vi "Cursor Release.vi"(6 "Control Ref Queue":T1, 8 "error in (no error)":errorcluster, 11 "2D Plot.lvclass in":refnum<class "2D Plot.lvclass">) -> (0 "error out":errorcluster, 3 "2D Plot.lvclass out":refnum<class "2D Plot.lvclass">)   [LabVIEW 2017, in "2D Plot.lvclass"]
uses:
  <vilib>/Math Plots/2D Math Plots/2D Plot/2D Plot/2D Plot.lvclass
  <vilib>/Math Plots/2D Math Plots/2D Plot/Action String/2DMathPlot Ctrl Act Queue.ctl
  <vilib>/Math Plots/2D Math Plots/2D Plot/Action String/2DMathPlot Ctrl Act Cluster.ctl
  <vilib>/Math Plots/2D Math Plots/2D Plot/Action String/2DMathPlot State Class.ctl
  <vilib>/Math Plots/2D Math Plots/2D Plot/2D Plot/2D Plot.lvclass/2D Plot.ctl
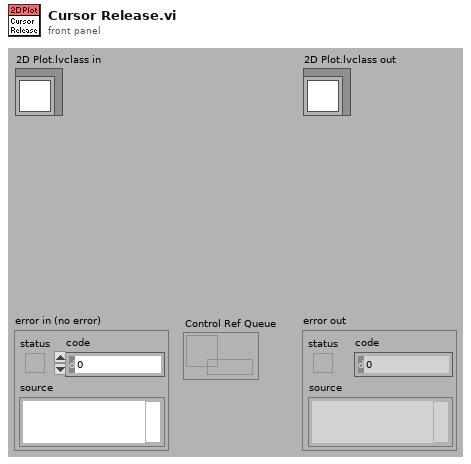
[diagram p1: front panel]
types:
  T1 = typedef "2DMathPlot Ctrl Act Queue.ctl" = refnum<queue>
  T2 = typedef "2DMathPlot Ctrl Act Cluster.ctl" = cluster{"Plot Area Ref":refnum<vi>, "Z Axis Ref":refnum<vi>, "Legend Ref":refnum<vi>, "XControl Ref":refnum<vi>, "Facade Ref":refnum<vi>, "Display State Change Class":T3}
  T3 = typedef "2DMathPlot State Class.ctl" = enum16{"Update All (Undo)", "Update General", "Update Appearance", "Update Format", "Update Scale", "Update Marker", "Update Cursor", "None"}
  T4 = typedef "LVAnnotationListTypeDef.ctl" = cluster{"Name":string, "Color":u32, "Style":u8, "Point Style":u8, "Name Visible":bool, "Allow Drag":bool, "Annotation Mode":u32, "Plot":i32, "Index":i32, "Position":cluster{"X":dbl, "Y":dbl}, "X Scale":u32, "Y Scale":u32, "Show Arrow":bool, "Lock Name":bool, "Plot Area":i32, "Label Offset":cluster{"X":dbl, "Y":dbl}}[]
  T5 = typedef "LVCursorListTypeDef.ctl" = cluster{"Name":string, "Color":u32, "Style":u8, "Point Style":u8, "Name Visible":bool, "Allow Drag":bool, "Cursor Mode":u32, "Plot":i32, "Index":i32, "Position":cluster{"X":dbl, "Y":dbl}, "X Scale":u32, "Y Scale":u32, "Watch Plots":i32[], "Watch All Plots":bool, "Plot Area":i32, "Label Offset":cluster{"X":dbl, "Y":dbl}}[]
  T6 = cluster{"Cursor Selection Color":u32, "Line Style":u8, "Line Width":u8, "Visible":bool}
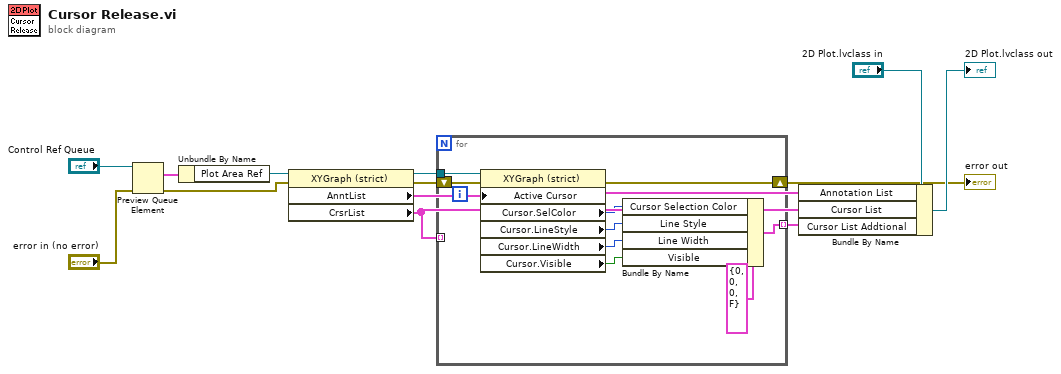
[diagram p0: block diagram]
diagram:
  n1 = Preview Queue Element(queue="Control Ref Queue", error in (no error)="error in (no error)") -> (element=w7:T2, error out=w8:errorcluster)  [unwired: 3 out]
  n2 = Unbundle By Name(w7) -> ("Plot Area Ref"=w10:refnum<vi>)
  n3 = property class="XYGraph (strict)"(reference=w10, error in=w8) -> (reference out=w6:refnum<vi>, error out=w5:errorcluster, "AnntList"=w1:T4, "CrsrList"=w2:T5)
  n4 = for {
    tunnel: w6 -> [w23]
    tunnel: w2 -> [_] mode=indexing
    shift-right: [w20] -> w4
    shift-left: w5 -> [w21]
    tunnel: [w14] -> w3 mode=indexing
    i -> [w22]
    n5 = property class="XYGraph (strict)"(reference=w23, error in=w21, "Active Cursor"=w22) -> (error out=w20:errorcluster, "Cursor.SelColor"=w18:u32, "Cursor.LineStyle"=w17:u8, "Cursor.LineWidth"=w16:u8, "Cursor.Visible"=w15:bool)  [unwired: 1 out]
    n6 = Bundle By Name(cluster=T6 {"Cursor Selection Color"=0, "Line Style"=0, "Line Width"=0, "Visible"=FALSE} ("Rest Attribute"), "Cursor Selection Color"=w18, "Line Style"=w17, "Line Width"=w16, "Visible"=w15) -> (w14:T6)
  }
  "error out" <- w4
  n7 = Bundle By Name(cluster="2D Plot.lvclass in", "Annotation List"=w1, "Cursor List"=w2, "Cursor List Addtional"=w3) -> (→"2D Plot.lvclass out":refnum<class "2D Plot.lvclass">)
